vi "Test.vi"() -> ()   [LabVIEW 2022 SP3]
panel:
  in  "Project Path":path=path "E:/VI2String/Test Project/Test Project.lvproj"
  in  "Project String Files Root":path=path "E:/VI2String/test"
  in  "Create Captions":bool=TRUE
  in  "Export Diagram":bool=TRUE
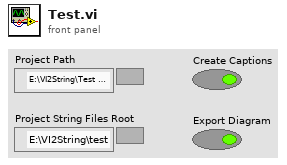
[diagram p1: front panel]
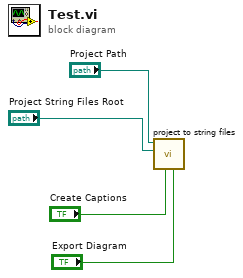
[diagram p0: block diagram]
diagram:
  n1 = call "project to string files.vi"("Export Diagram"="Export Diagram", "Create Captions"="Create Captions", "Project String Files Root"="Project String Files Root", "Project Path"="Project Path") -> ()  [unwired: 7 in, 1 out]
